vi "Read U8 External Payload.vi"(8 "error in (no error)":errorcluster, 9 "Timeout (ms)":i32, 10 "Data in":u8[](array[numeric]), 11 "CIFFIFO in":refnum<class "CIF_CIPC_Fifo_U8.lvclass">) -> (0 "error out":errorcluster, 1 "timed out?":bool, 2 "Data out":u8[](array[numeric]), 3 "CIFFIFO out":refnum<class "CIF_CIPC_Fifo_U8.lvclass">, 4 "Header":T1)   [LabVIEW 2021, in "CIF_CIPC_Fifo_U8.lvclass"]
doc: "Read the full payload bytes, including the encoded header. This is intended for advanced applications where the full buffer will be sent externally."
uses:
  CIF_CIPC_Fifo_U8.lvclass
  ChannelCommon/typedef/FIFO Header.ctl
  D:/dev/Packages/CIF_Channels_Core/src/CIFChannels/CIFChannels.lvclass
  D:/dev/Packages/CIF_Channels_Core/src/CIPC_Channels/CIF_CIPC_Chan/CIF_CIPC_Chn.lvclass
  CIFChannels/CIFChannels.lvclass/CIFChannels.ctl
  CIF_CIPC_Chan/CIF_CIPC_Chn.lvclass/CIF_CIPC_Chn.ctl
  CIF_CIPC_Fifo_U8.lvclass/CIF_CIPC_Fifo_U8.ctl
  <vilib>/CIF Foundation/CIF Utilities/Statistics/I64/Stats_I64_CIF_U.lvclass/Stats_I64_CIF_U.ctl
  CIFChannels/Accessors/Read FIFO Payload Length.vi
  CIFChannels/Accessors/Read FIFO Header.vi
  ChannelCommon/Utilities/Unflatten Header.vi
  SubVIs/Read Wrapper for Backpressure Support.vi
  CIFChannels/Accessors/Write FIFO Header.vi
  ChannelCommon/Utilities/Remove Header Bytes.vi
  CIFChannels/Utilities/Update Channel Benchmark.vi
  SubVIs/Core Read U8 FIFO.vi/e703c505-0034-46a9-8989-21c0de27793f.vi
  SubVIs/Core Read U8 FIFO.vi/768488f4-e6df-4560-a449-a64b33b49031.vi
  CIFChannels/Accessors/Read Channel State.vi
  CIFChannels/Accessors/Read Direction.vi
  <vilib>/CIF Foundation/CIF Utilities/DataTypes/Flatten Unflatten/Unflatten U64.vi
  <vilib>/CIF Foundation/CIF Utilities/DataTypes/Flatten Unflatten/Unflatten I64.vi
  ChannelCommon/Utilities/Add Error.vi
  CIF_CIPC_Chan/Accessors/Read CIPC Channel.vi
  SubVIs/Read Wrapper for Backpressure Support.vi/b5615cf0-cd7f-4476-b9a9-d6ef7628cc3b.vi
  CIF_CIPC_Chan/Accessors/Read Buffer Configuration.vi
  SubVIs/Read Wrapper for Backpressure Support.vi/6248fc70-cc83-4025-b778-a3221b95feac.vi
  CIFChannels/Accessors/Read FIFO Backpressure.vi
  <vilib>/CIF Foundation/CIF Utilities/Statistics/I64/X1 minus X0.vi
  <vilib>/CIF Foundation/CIF Utilities/Time/System Time/Get System Time.vi
  <vilib>/CIF Foundation/CIF CIPC/SubVIs/Wait For N Elements Available.vi
  <vilib>/CIF Foundation/CIF CIPC/SubVIs/Get Element Read Position.vi
  <vilib>/CIF Foundation/CIF CIPC/SubVIs/Check Error.vi
  <vilib>/CIF Foundation/CIF CIPC/SubVIs/Get dll Path.vi
  <vilib>/CIF Foundation/CIF CIPC/SubVIs/Set Element Read Position.vi
  SubVIs/Read Wrapper for Backpressure Support.vi/6248fc70-cc83-4025-b778-a3221b95feac.vi/331f6ecb-7ec4-4931-b93d-4fbd8d66a851.vi
  SubVIs/Read Wrapper for Backpressure Support.vi/6248fc70-cc83-4025-b778-a3221b95feac.vi/5ce0d4cf-f921-42ba-b14c-c90f7f7611e4.vi
  <vilib>/CIF Foundation/CIF Utilities/Statistics/I64/X1 minus X0.vi/dfabcf33-0dbc-4041-80a5-3dc0c86d2989.vi
  <vilib>/CIF Foundation/CIF Utilities/Time/System Time/LabVIEW Time to TAI Time.vi
  <vilib>/CIF Foundation/CIF CIPC/SubVIs/Notify Of New Write.vi
  <vilib>/CIF Foundation/CIF CIPC/SubVIs/Get Element Write Position.vi
  <vilib>/CIF Foundation/CIF Utilities/Statistics/I64/X1 minus X0.vi/dfabcf33-0dbc-4041-80a5-3dc0c86d2989.vi/9eb60a9a-770f-4d2d-8b3f-8465c267ecc9.vi
  <vilib>/CIF Foundation/CIF CIPC/SubVIs/Check Error Core.vi
  <vilib>/CIF Foundation/CIF CIPC/SubVIs/Get Element Info Variant.vi
  ChannelCommon/Utilities/Add Error Core.vi
  ChannelCommon/ChannelCommon.lvlib
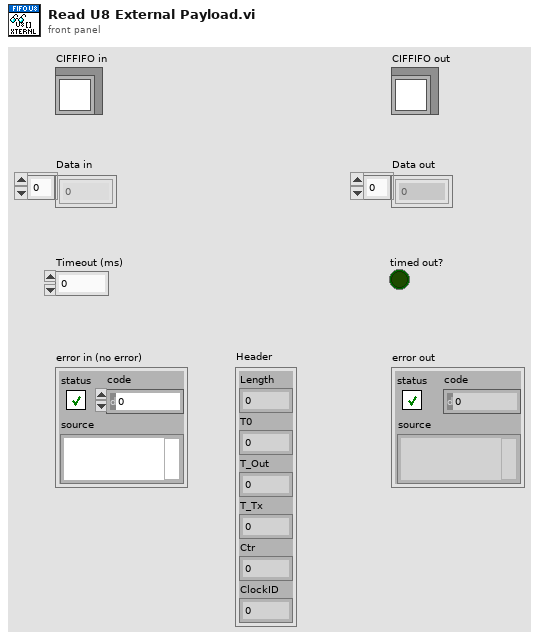
[diagram p1: front panel]
types:
  T1 = typedef "ChannelCommon.lvlib/FIFO Header.ctl" = cluster{"Length":u64, "T0":i64, "T_Out":i64, "T_Tx":i64, "Ctr":u64, "ClockID":u8}
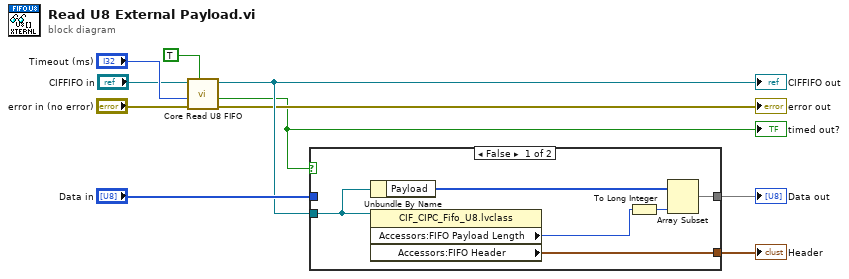
[diagram p0: block diagram]
diagram:
  n1 = call "Core Read U8 FIFO.vi"("Include Header"=TRUE, "error in (no error)"="error in (no error)", "Timeout (ms)"="Timeout (ms)", "CIFFIFO in"="CIFFIFO in") -> ("error out"=→"error out":errorcluster, "timed out?"=w2:bool, "CIFFIFO out"=w4:refnum<class "CIF_CIPC_Fifo_U8.lvclass">)  [unwired: 5 in]
  "timed out?" <- w2
  "CIFFIFO out" <- w4
  n2 = case shown="False" w2 {
    tunnel: w4 -> [w16 _]
    tunnel: [w14 w17] -> w6
    tunnel: [w13 _] -> w7
    tunnel: "Data in" -> [_ w17]
    frame False {
      n3 = Unbundle By Name(w16) -> ("Payload"=w15:u8[])
      n4 = property class="CIF_CIPC_Fifo_U8.lvclass"(reference=w16) -> ("Accessors:FIFO Payload Length"=w11:u64, "Accessors:FIFO Header"=w13:T1)  [unwired: 1 in, 2 out]
      n5 = To Long Integer(number=w11) -> (32bit integer=w12:i32)
      n6 = Array Subset(array=w15, length=w12) -> (w14:u8[])  [unwired: 1 in]
    }
    frame True {
    }
  }
  "Header" <- w7
  "Data out" <- w6
